vi "SAT.vi"() -> ()   [LabVIEW 2015]
uses:
  <vilib>/LabVIEW Targets/FPGA/cRIO/shared/nicrio_ModuleControls/nicrio_cRIO-9234_DataRatesRing2.ctl
  <vilib>/userdefined/High Color/nirio_resource_hc.ctl
  <vilib>/FPGAPlugInAG/cRIO-9031/niLvFpga_Open_cRIO-9031.vi
  <vilib>/FPGAPlugInAG/cRIO-9031/niLvFpga_Run_cRIO-9031.vi
  <vilib>/Utility/error.llb/Error Cluster From Error Code.vi
  <vilib>/rvi/errors/niLvFpgaAdjustHostInterfaceError.vi
  <vilib>/rvi/interface/common/niFpgaWaitOnOcc.vi
  <vilib>/FPGAPlugInAG/cRIO-9031/niLvFpga_Reset_cRIO-9031.vi
  <vilib>/rvi/interface/nirviOpenFPGA/nirviOpenFPGA.xnode
  WRDArabia_FPGATarget_FPGA8a2wsBIdirec_rZEOcJD8nrk.lvbitx
  <vilib>/rvi/interface/nirviMethod/nirviMethod.xnode
  <vilib>/rvi/interface/nirviReadWriteControl/nirviReadWriteControl.xnode
  <vilib>/FPGAPlugInAG/cRIO-9031/niLvFpga_ConfigureFifo_cRIO-9031.vi
  <vilib>/rvi/errors/niLvFpgaMergeErrorWithErrorCode.vi
  <vilib>/FPGAPlugInAG/cRIO-9031/niLvFpga_StartFifo_cRIO-9031.vi
  NiFpgaLv.dll
  <vilib>/FPGAPlugInAG/cRIO-9031/niLvFpga_ReadFifo_cRIO-9031.vi
  <vilib>/FPGAPlugInAG/cRIO-9031/niLvFpga_StopFifo_cRIO-9031.vi
panel:
  in  "STOP":bool
  out "Buffer Underflow":bool
  out "Buffer Overflow":bool
  out "Numeric":i32
  in  "Rate frequency (Hz)":dbl=25600.0
  in  "Data Rate":T1=2 items=["51.200 kS/s (NI 9234)"=1, "25.600 kS/s (NI 9234)"=2, "17.067 kS/s (NI 9234)"=3, "12.800 kS/s (NI 9234)"=4, "10.240 kS/s (NI 9234)"=5, "8.533 kS/s (NI 9234)"=6, "7.314 kS/s (NI 9234)"=7, "6.400 kS/s (NI 9234)"=8, "5.689 kS/s (NI 9234)"=9, "5.120 kS/s (NI 9234)"=10, "4.654 kS/s (NI 9234)"=11, "4.267 kS/s (NI 9234)"=12, "3.938 kS/s (NI 9234)"=13, "3.657 kS/s (NI 9234)"=14, "3.413 kS/s (NI 9234)"=15, "3.200 kS/s (NI 9234)"=16, "3.012 kS/s (NI 9234)"=17, "2.845 kS/s (NI 9234)"=18, "2.695 kS/s (NI 9234)"=19, "2.560 kS/s (NI 9234)"=20, "2.438 kS/s (NI 9234)"=21, "2.328 kS/s (NI 9234)"=22, "2.226 kS/s (NI 9234)"=23, "2.133 kS/s (NI 9234)"=24, "2.048 kS/s (NI 9234)"=25, "1.969 kS/s (NI 9234)"=26, "1.896 kS/s (NI 9234)"=27, "1.829 kS/s (NI 9234)"=28, "1.765 kS/s (NI 9234)"=29, "1.707 kS/s (NI 9234)"=30, "1.652 kS/s (NI 9234)"=31]
  out "Chassis \nTemperature":dbl
  out "error out":errorcluster
  in  "Tab Control":enum32{"Wheel Sensor", "Accelerometer"}(tab)
  out "Waveform Graph":dbl[](graph)
  out "Acc":sgl[][](graph)
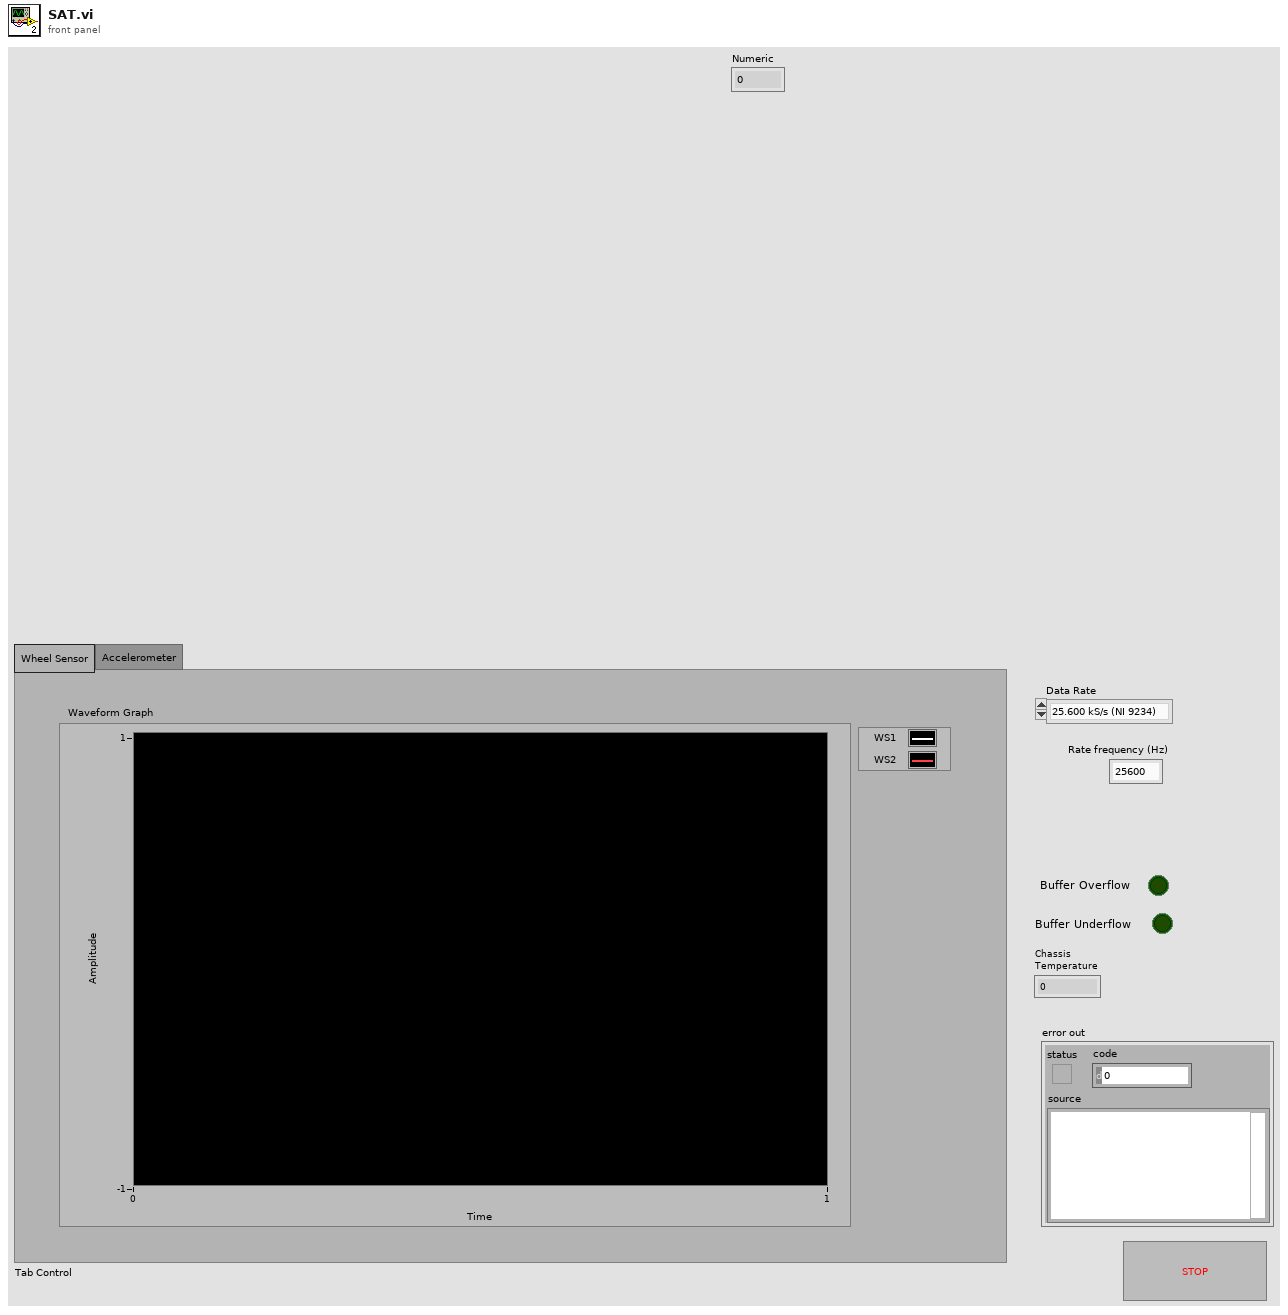
[diagram p1: front panel]
types:
  T1 = typedef "nicrio_cRIO-9234_DataRatesRing2.ctl" = u8
  T2 = typedef "nirio_resource_hc.ctl" = tag
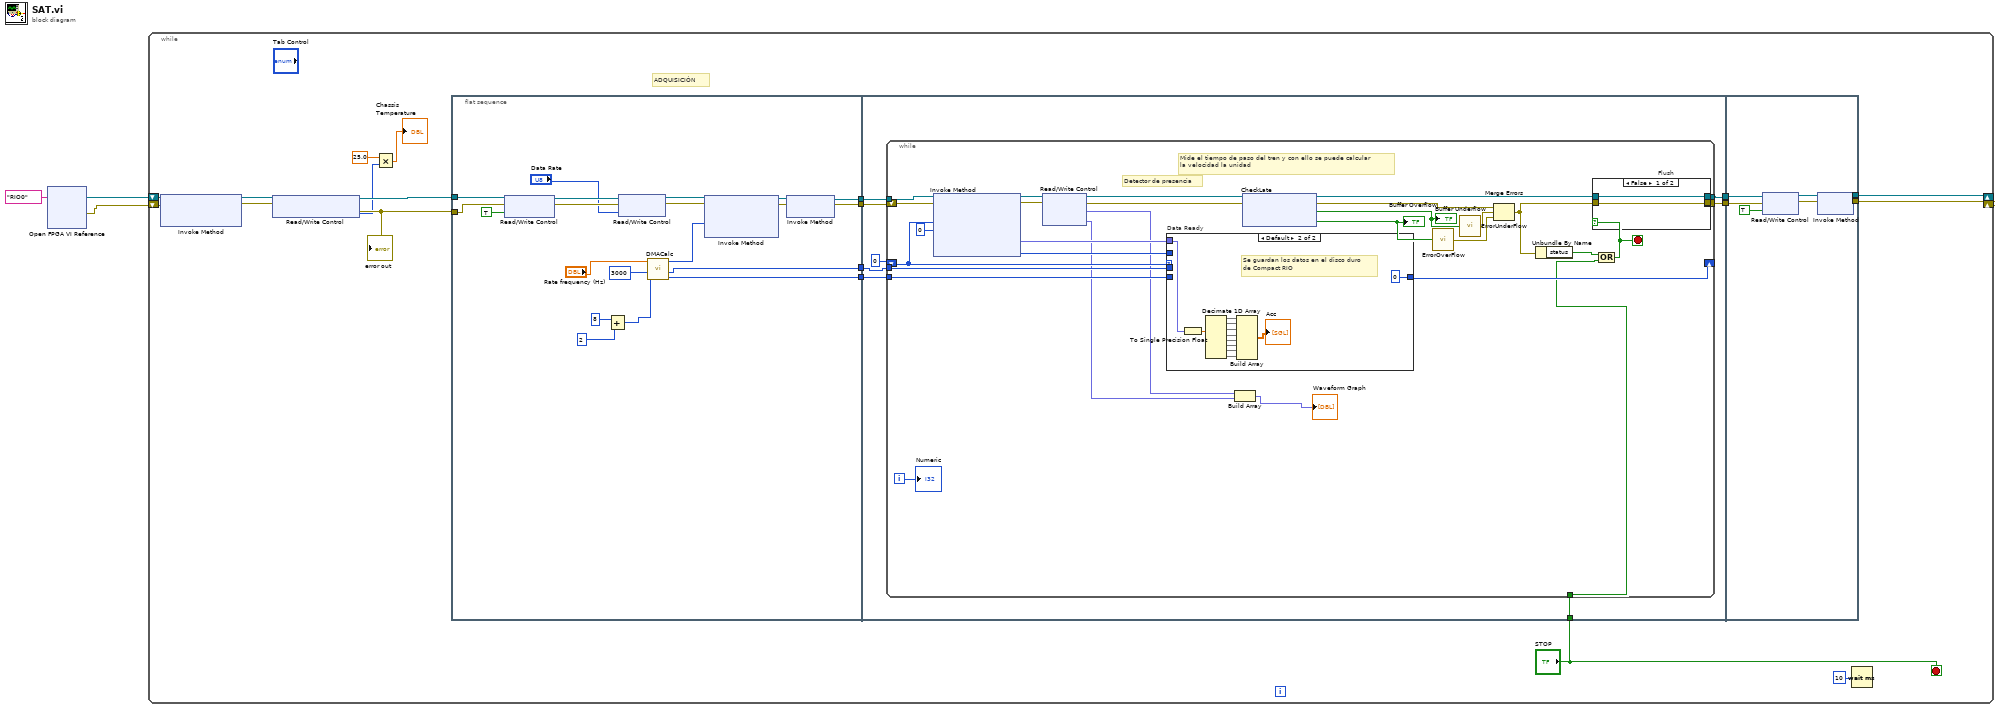
[diagram p0: block diagram]
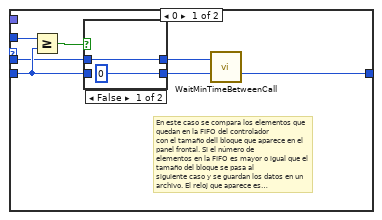
[diagram p2: hidden frame]
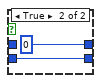
[diagram p3: hidden frame]
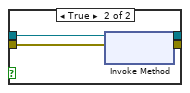
[diagram p4: hidden frame]
diagram:
  n1 = xnode "Open FPGA VI Reference"("resource name"=T2 "RIO0") -> ("FPGA VI Reference Out"=w2:refnum<k20>, "error out"=w1:errorcluster)  [unwired: 1 in]
  n2 = while {
    shift-right: [w18] -> _
    shift-left: w2 -> [w16]
    shift-right: [w21] -> _
    shift-left: w1 -> [w15]
    stop <- "STOP" stop-if-true
    # "ADQUISICIÓN"
    n3 = xnode "Invoke Method"("FPGA VI Reference In"=w16, "error in"=w15) -> ("FPGA VI Reference Out"=w17:refnum<k20>, "error out"=w14:errorcluster)  [unwired: 1 in]
    n4 = xnode "Read/Write Control"("FPGA VI Reference In"=w17, "error in"=w14) -> ("FPGA VI Reference Out"=w20:refnum<k20>, "error out"=w19:errorcluster, "Chassis Temperature"=w6:i16)
    "error out" <- w19
    n5 = Multiply(x=25.0, y=w6) -> (x*y=→"Chassis \nTemperature":dbl)
    n6 = flat-sequence {
      tunnel: w19 -> [w30]
      tunnel: w20 -> [w31]
      tunnel: [w39] -> w13
      tunnel: [w38] -> w12
      tunnel: [w37] -> w11
      tunnel: [w36] -> w10
      tunnel: [w49] -> w9
      tunnel: [w48] -> w8
      tunnel: w13 -> [w47]
      tunnel: w12 -> [w46]
      tunnel: w11 -> [w45]
      tunnel: w10 -> [w44]
      tunnel: "STOP" -> [w43]
      tunnel: w9 -> [w109]
      tunnel: w8 -> [w108]
      tunnel: [w113] -> w21
      tunnel: [w114] -> w18
      frame #0 {
        n7 = xnode "Read/Write Control"("FPGA VI Reference In"=w31, "error in"=w30, "Fotocélula"=TRUE ("Adquirir")) -> ("FPGA VI Reference Out"=w29:refnum<k20>, "error out"=w28:errorcluster)
        n8 = Add(x=u32 8, y=u32 2) -> (x+y=w25:u32)
        n9 = xnode "Read/Write Control"("FPGA VI Reference In"=w29, "error in"=w28, "Data Rate"="Data Rate") -> ("FPGA VI Reference Out"=w35:refnum<k20>, "error out"=w34:errorcluster)
        n10 = call "DMACalc.vi"("Number of Channels"=w25, "Number of Samples"=u32 3000, "Rate (Hz)"="Rate frequency (Hz)") -> ("Block Size"=w36:u32, "Time to Acquire Block (ms)"=w37:i32, "Host Buffer Size"=w40:u32)  [unwired: 6 in]
        n11 = xnode "Invoke Method"("FPGA VI Reference In"=w35, "error in"=w34, "Requested Depth"=w40) -> ("FPGA VI Reference Out"=w42:refnum<k20>, "error out"=w41:errorcluster)  [unwired: 1 out]
        n12 = xnode "Invoke Method"("FPGA VI Reference In"=w42, "error in"=w41) -> ("FPGA VI Reference Out"=w39:refnum<k20>, "error out"=w38:errorcluster)
      }
      frame #1 {
        n13 = while "Data Acquisition" {
          tunnel: w47 -> [w70]
          shift-right: [w77] -> _
          shift-left: u32 0 ("t") -> [w73]
          tunnel: w45 -> [w78]
          tunnel: w44 -> [w76]
          shift-right: [w79] -> w48
          shift-left: w46 -> [w69]
          tunnel: [w74] -> w49
          tunnel: w43 -> [w58]
          i -> [w59]
          stop <- w75 stop-if-true
          # "Detector de presencia"
          # "Mide el tiempo de paso del tren y con ello se puede calcular\nla velocidad la unidad"
          n14 = xnode "Invoke Method"("FPGA VI Reference In"=w70, "error in"=w69, "Number of Elements"=w73, "Timeout (ms)"=0) -> ("FPGA VI Reference Out"=w57:refnum<k20>, "error out"=w56:errorcluster, "Data"=w68:fxp<+/-,24,4>[], "Elements Remaining"=w71:u32)
          n15 = xnode "Read/Write Control"("FPGA VI Reference In"=w57, "error in"=w56) -> ("FPGA VI Reference Out"=w55:refnum<k20>, "error out"=w54:errorcluster, "WhlCnt1"=w53:fxp<+/-,24,-4>, "WhlCnt2"=w52:fxp<+/-,24,-4>)
          n16 = case "Data Ready" shown="Default" w73 {
            tunnel: w78 -> [w82 _]
            tunnel: [w81 u32 0 ("t")] -> w77
            tunnel: w76 -> [w83 _]
            tunnel: w71 -> [w80 _]
            tunnel: w68 -> [_ w100]
            frame 0 {
              # "En este caso se compara los elementos que quedan en la FIFO del controlador\ncon el tamaño dell bloque que aparece en el panel frontal. Si el número de\nelementos en la FIFO es mayor o igual que el tamaño del bloque se pasa al\nsiguiente caso y se guardan los datos en un archivo. El reloj que aparece es\nuna espera para no consumir recursos."
              n17 = Greater Or Equal?(x=w80, y=w83) -> (x >= y?=w84:bool)
              n18 = case shown="False" w84 {
                tunnel: [u32 0 ("Block Size") w88] -> w81
                tunnel: [w87 0 ("t")] -> w85
                tunnel: w82 -> [w87 _]
                tunnel: w83 -> [_ w88]
                frame False {
                }
                frame True {
                }
              }
              n19 = call "WaitMinTimeBetweenCall.vi"("Minimum ms between calls"=w85) -> ()  [unwired: 2 in]
            }
            frame Default {
              # "Se guardan los datos en el disco duro\nde Compact RIO"
              n20 = To Single Precision Float(number=w100) -> (single precision float=w93:sgl[])
              n21 = Decimate 1D Array(w93) -> (w99:sgl[], w95:sgl[], w96:sgl[], w97:sgl[], w98:sgl[], w94:sgl[], w92:sgl[], w91:sgl[])
              n22 = Build Array(w99, w95, w96, w97, w98, w94, w92, w91) -> (→"Acc":sgl[][])
            }
          }
          n23 = Build Array(w53, w52) -> (→"Waveform Graph":fxp<+/-,24,-4>[])
          n24 = xnode ("CheckLate")("FPGA VI Reference In"=w55, "error in"=w54) -> ("FPGA VI Reference Out"=w60:refnum<k20>, "error out"=w64:errorcluster, "Buffer Underflow"=w65:bool, "Buffer Overflow"=w66:bool)
          "Buffer Underflow" <- w65
          "Buffer Overflow" <- w66
          n25 = call "ErrorOverFlow.vi"("Buffer Overflow"=w66) -> ("error out"=w62:errorcluster)
          n26 = call "ErrorUnderFlow.vi"("Buffer Overflow"=w65) -> ("error out"=w63:errorcluster)
          n27 = Merge Errors(w64, w63, w62) -> (w61:errorcluster)
          n28 = Unbundle By Name(w61) -> ("status"=w67:bool)
          n29 = Compound Arithmetic op=OR(w67, w58) -> (w75:bool)
          n30 = case "Flush" shown="False" w75 {
            tunnel: w60 -> [w102 w107]
            tunnel: w61 -> [w103 w106]
            tunnel: [w103 w105] -> w79
            tunnel: [w102 w104] -> w74
            frame False {
            }
            frame True {
              n31 = xnode "Invoke Method"("FPGA VI Reference In"=w107, "error in"=w106) -> ("FPGA VI Reference Out"=w104:refnum<k20>, "error out"=w105:errorcluster)
            }
          }
          "Numeric" <- w59
        }
      }
      frame #2 {
        n32 = xnode "Read/Write Control"("FPGA VI Reference In"=w109, "error in"=w108, "Stop"=TRUE ("stop")) -> ("FPGA VI Reference Out"=w112:refnum<k20>, "error out"=w111:errorcluster)
        n33 = xnode "Invoke Method"("FPGA VI Reference In"=w112, "error in"=w111) -> ("FPGA VI Reference Out"=w114:refnum<k20>, "error out"=w113:errorcluster)
      }
    }
    n34 = Wait (ms)(milliseconds to wait=u32 10) -> ()  [unwired: 1 out]
  }
